vi "Write TCP Message.vi"(8 "error in (no error)":errorcluster, 10 "Message (string)":string, 11 "TCP Network Connection in":refnum<k5>) -> (0 "error out":errorcluster, 3 "TCP Network Connection out":refnum<k5>)   [LabVIEW 2019, in "TimingDRV System Explorer.lvlib"]
uses:
  TimingDRV System Explorer.lvlib
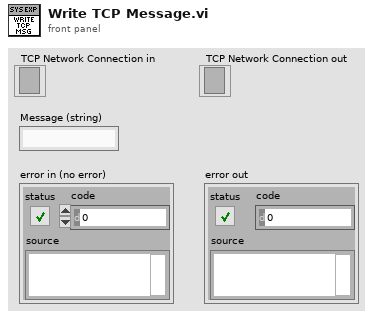
[diagram p1: front panel]
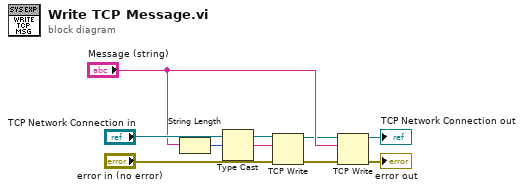
[diagram p0: block diagram]
diagram:
  n1 = String Length(string="Message (string)") -> (length=w2:i32)
  n2 = Type Cast(x=w2) -> (*(type *) &x=w1:string)  [unwired: 1 out]
  n3 = TCP Write(connection ID="TCP Network Connection in", data in=w1, error in (no error)="error in (no error)") -> (connection ID out=w3:refnum<k5>, error out=w5:errorcluster)  [unwired: 2 out]
  n4 = TCP Write(connection ID=w3, data in="Message (string)", error in (no error)=w5) -> (connection ID out=→"TCP Network Connection out":refnum<k5>, error out=→"error out":errorcluster)  [unwired: 2 out]
